vi "Init Execution.vi"(8 "error in":errorcluster, 11 "PAS Control in":refnum<class "PAS Control.lvclass">) -> (0 "error out":errorcluster, 2 "Stop Event":refnum<user-event>, 3 "PAS Control out":refnum<class "PAS Control.lvclass">)   [LabVIEW 2012, in "PAS Control.lvclass"]
uses:
  PAS Control.lvclass
  Reusable/GUI/GUI.lvclass
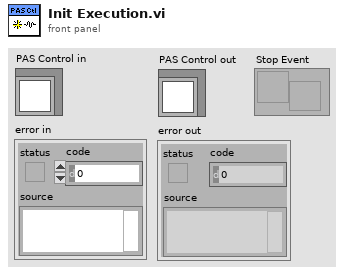
[diagram p1: front panel]
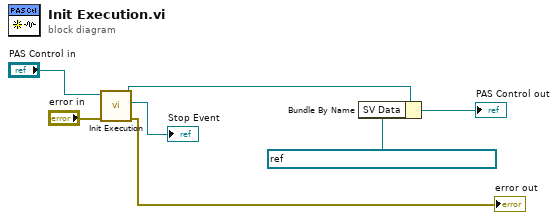
[diagram p0: block diagram]
diagram:
  n1 = call-parent "Init Execution.vi"("error in"="error in", "GUI in"="PAS Control in") -> ("error out"=→"error out":errorcluster, "Stop Event"=→"Stop Event":refnum<user-event>, "GUI out"=w4:refnum<class "PAS Control.lvclass">)  [unwired: 7 in]
  n2 = Bundle By Name(cluster=w4, "SV Data"=refnum<k21> "ni.var.psp://rt pxi target/PAS_Var/Data" ("shared variable refnum in")) -> (→"PAS Control out":refnum<class "PAS Control.lvclass">)
